vi "Handle.vi"(8 "Error In":errorcluster, 9 "Action":string, 10 "Values":dbl[](array[numeric]), 11 "reference in":refnum<class "AdditionHandler.lvclass">) -> (0 "Error Out":errorcluster, 2 "Return(DBL)":dbl, 3 "reference in":refnum<class "AdditionHandler.lvclass">)   [LabVIEW 2020, in "AdditionHandler.lvclass"]
uses:
  AdditionHandler.lvclass
  C:/Projects/DesignPatterns/ChainOfResponsibilityPattern/BaseHandler_class/BaseHandler.lvclass
  IHandler_interface/IHandler.lvclass
  BaseHandler_class/BaseHandler.lvclass
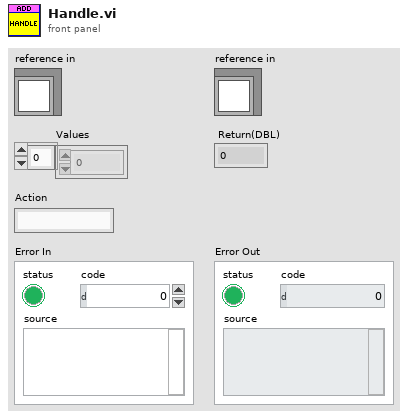
[diagram p1: front panel]
types:
  T1 = typedef "BaseHandler.lvclass/ObjectAttributes.ctl" = cluster{"_nextInLine":refnum<class "IHandler.lvclass">}
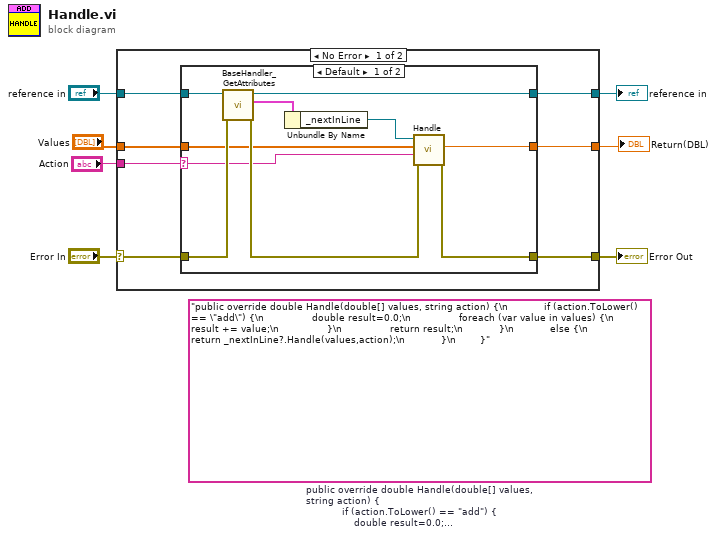
[diagram p0: block diagram]
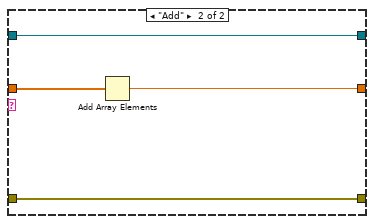
[diagram p2: hidden frame]
diagram:
  (unwired) "public override double Handle(double[] values, string action) {\n            if (action.ToLower() == \"add\") {\n                double result=0.0;\n                foreach (var value in values) {\n                    result += value;\n                }\n                return result;\n            }\n            else {\n                return _nextInLine?.Handle(values,action);\n            }\n        }"  # public override double Handle(double[] values, string action) {             if (action.ToLower() == "add") {                 double result=0.0;                 foreach (var value in values) {                     result += value;                 }                 return result;             }             else {                 return _nextInLine?.Handle(values,action);             }         }
  n1 = case shown="No Error" "Error In" {
    selector: "Error In" -> [w13 w30]
    tunnel: [w11 w30] -> w6
    tunnel: [w12 w29] -> w4
    tunnel: "reference in" -> [w14 w29]
    tunnel: "Action" -> [w10 _]
    tunnel: "Values" -> [w9 _]
    tunnel: [w8 _] -> w1
    frame No Error {
      n2 = case shown="Default" w10 {
        selector: w10 -> [w17 _]
        tunnel: w14 -> [w24 w28]
        tunnel: w13 -> [w23 w27]
        tunnel: [w22 w28] -> w12
        tunnel: [w19 w27] -> w11
        tunnel: w9 -> [w18 w26]
        tunnel: [w16 w25] -> w8
        frame Default {
          n3 = call "BaseHandler_GetAttributes.vi"("error in (no error)"=w23, "reference in"=w24) -> ("error out"=w20:errorcluster, "Data"=w21:T1, "reference out"=w22:refnum<class "AdditionHandler.lvclass">)  [unwired: 6 in, 1 out]
          n4 = Unbundle By Name(w21) -> ("_nextInLine"=w15:refnum<class "IHandler.lvclass">)
          n5 = call-dynamic "Handle.vi"("Error In"=w20, "Action"=w17, "Values"=w18, "object in"=w15) -> ("Error Out"=w19:errorcluster, "Return(DBL)"=w16:dbl)  [unwired: 5 in, 1 out]
        }
        frame "Add" {
          n6 = Add Array Elements(numeric array=w26) -> (sum=w25:dbl)
        }
      }
    }
    frame Error {
    }
  }
  "Error Out" <- w6
  "reference in" <- w4
  "Return(DBL)" <- w1
